vi "Main.vi"() -> ()   [LabVIEW 2019]
uses:
  support/Panel Selector (Radio Button).ctl
  support/Main_States.ctl
  support/Main_StateData.ctl
  Common Components/Hardware/DMM/DMM.lvclass
  Common Components/Hardware/FGEN/Function Generator.lvclass
  Common Components/Hardware/Scope/Scope.lvclass
panel:
  in  "Panel Selector (Radio Button)":T1
  # "Componentized Demo"
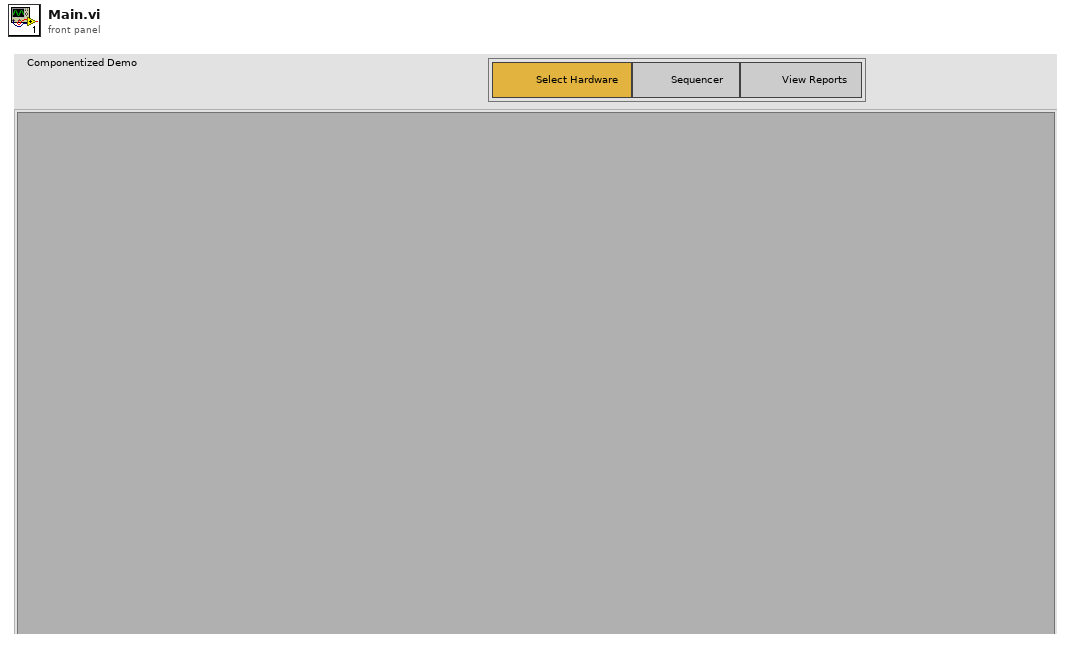
[diagram p1: front panel]
types:
  T1 = typedef "Panel Selector (Radio Button).ctl" = enum32{"Select HW", "Sequencer", "View Reports"}
  T2 = typedef "Main_StateData.ctl" = cluster{"Subpanel VI refs":refnum<vi>[]}
  T3 = typedef "Main_States.ctl" = enum16{"Initialize", "Wait for Event", "Shutdown"}
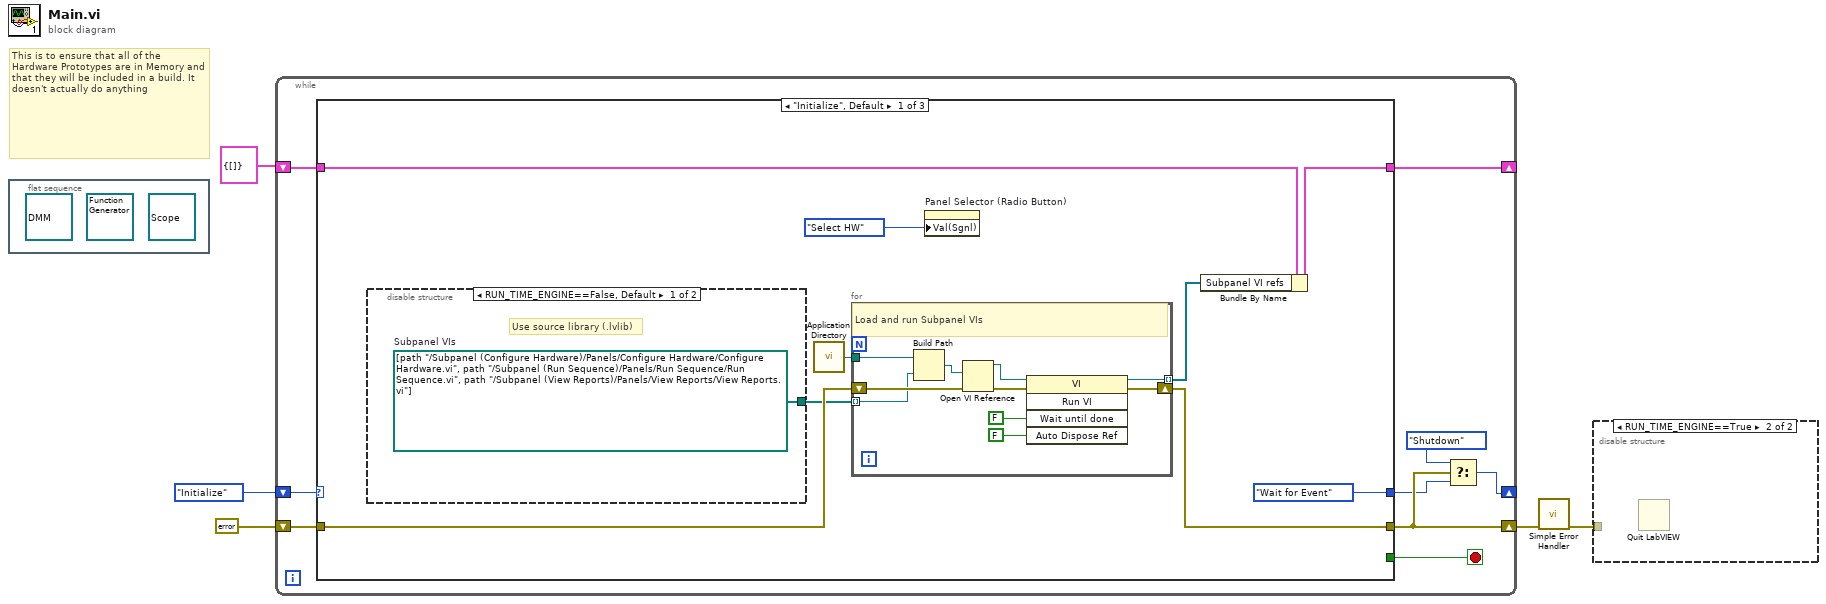
[diagram p0: block diagram]
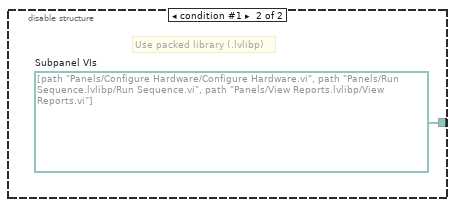
[diagram p3: hidden frame]
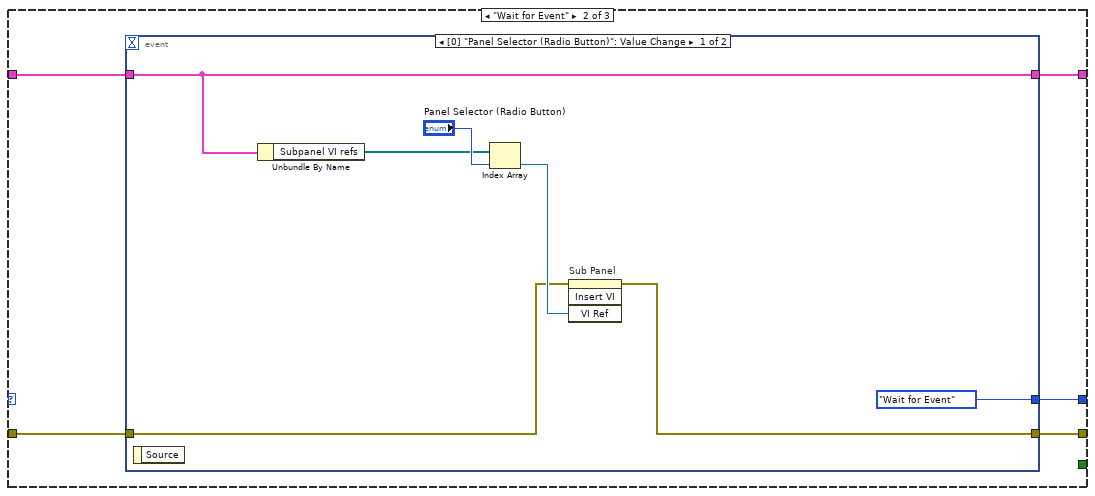
[diagram p4: hidden frame]
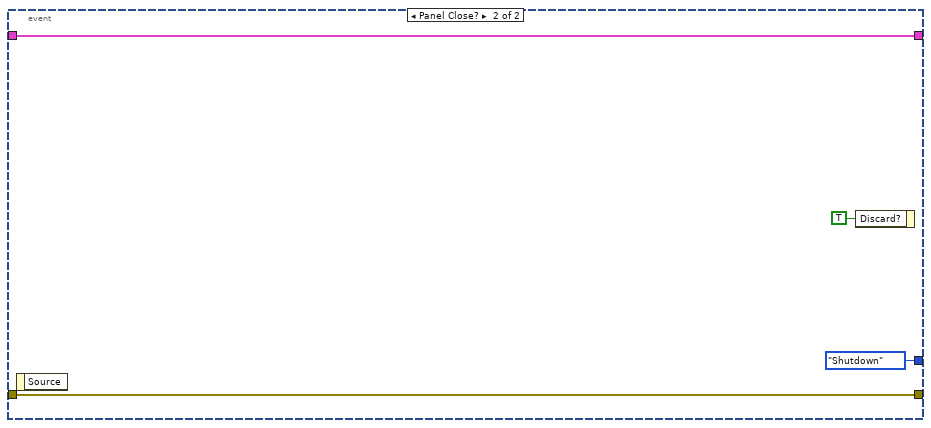
[diagram p5: hidden frame]
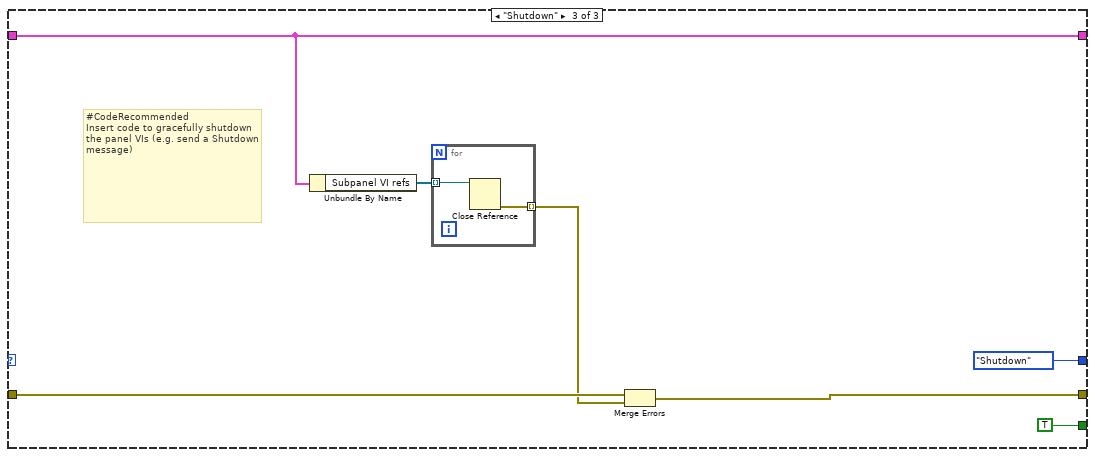
[diagram p6: hidden frame]
diagram:
  # "This is to ensure that all of the Hardware Prototypes are in Memory and that they will be included in a build. It doesn't actually do anything"
  n1 = flat-sequence {
    frame #0 {
      (unwired) refnum<class "Scope.lvclass"> refnum ("Hardware.lvlib:Scope.lvclass")
      (unwired) refnum<class "Function Generator.lvclass"> refnum ("Hardware.lvlib:Function Generator.lvclass")
      (unwired) refnum<class "DMM.lvclass"> refnum ("Hardware.lvlib:DMM.lvclass")
    }
  }
  n2 = while {
    shift-right: [w6] -> _
    shift-left: Main_States."Initialize" -> [w14]
    shift-right: [w9] -> w2
    shift-left: errorcluster {"status"=FALSE, "code"=0, "source"=""} ("error constant") -> [w12]
    shift-right: [w10] -> _
    shift-left: T2 {"Subpanel VI refs"=[]} ("Main_StateData") -> [w11]
    stop <- w13 stop-if-true
    n3 = case shown="\"Initialize\", Default" w14 {
      tunnel: [Main_States."Wait for Event" w40 Main_States."Shutdown"] -> w8
      tunnel: [_ _ TRUE] -> w13
      tunnel: w12 -> [w21 w37 w56]
      tunnel: [w20 w36 w53] -> w9
      tunnel: w11 -> [w18 w39 w55]
      tunnel: [w17 w38 w55] -> w10
      frame "Initialize", Default {
        n4 = disable-structure shown="RUN_TIME_ENGINE==False, Default" {
          disable-tunnel: [w24 w25] -> w19
          frame condition #0 (active) {
            w24 = path[] [path "../Subpanel (Configure Hardware)/Panels/Configure Hardware/Configure Hardware.vi", path "../Subpanel (Run Sequence)/Panels/Run Sequence/Run Sequence.vi", path "../Subpanel (View Reports)/Panels/View Reports/View Reports.vi"]  # Subpanel VIs
            # "Use source library (.lvlib)"
          }
          frame condition #1 {
            w25 = path[] [path "Panels/Configure Hardware/Configure Hardware.vi", path "Panels/Run Sequence.lvlibp/Run Sequence.vi", path "Panels/View Reports.lvlibp/View Reports.vi"]  # Subpanel VIs
            # "Use packed library (.lvlibp)"
          }
        }
        n5 = call <vilib>:"Application Directory.vi"() -> ("Application Directory"=w23:path)
        n6 = for {
          tunnel: [w31] -> w16 mode=indexing
          shift-right: [w29] -> w20
          shift-left: w21 -> [w30]
          tunnel: w23 -> [w28]
          tunnel: w19 -> [w26] mode=indexing
          # "Load and run Subpanel VIs"
          n7 = Build Path(base path=w28, name or relative path=w26) -> (appended path=w27:path)
          n8 = Open VI Reference(vi path=w27, error in (no error)=w30) -> (vi reference=w32:refnum<vi>, error out=w33:errorcluster)  [unwired: 4 in]
          n9 = invoke class="VI" method="Run VI"(reference=w32, error in=w33, "Wait until done"=FALSE ("Wait Until Done"), "Auto Dispose Ref"=FALSE ("Auto Dispose Reference")) -> (reference out=w31:refnum<vi>, error out=w29:errorcluster)  [unwired: 1 in, 3 out]
        }
        n10 = property on="Panel Selector (Radio Button)" class="RadioBtnsControl (strict)"("Val(Sgnl)"=Panel_Selector_(Radio_Button)."Select HW" ("Value (Signaling)")) -> ()  [unwired: 2 in, 2 out]
        n11 = Bundle By Name(cluster=w18, "Subpanel VI refs"=w16) -> (w17:T2)
      }
      frame "Wait for Event" {
        n12 = event shown="[0] \"Panel Selector (Radio Button)\": Value Change" {
          selector: _ -> [_ _]
          dyn-events: _ -> [_ _]
          timeout: _ -> [_ _]
          tunnel: [Main_States."Wait for Event" Main_States."Shutdown"] -> w40
          tunnel: w39 -> [w45 w49]
          tunnel: [w45 w49] -> w38
          tunnel: w37 -> [w42 w48]
          tunnel: [w41 w48] -> w36
          event Value Change {
            n13 = event-data() -> ()  [unwired: 1 in, 1 out]
            n14 = Unbundle By Name(w45) -> ("Subpanel VI refs"=w44:refnum<vi>[])
            n15 = Index Array(array=w44, index="Panel Selector (Radio Button)") -> (element=w43:refnum<vi>)
            n16 = invoke on="Sub Panel" class="SubPnl" method="Insert VI"(error in=w42, "VI Ref"=w43) -> (error out=w41:errorcluster)  [unwired: 2 in, 3 out]
          }
          event Panel Close? {
            n17 = event-data() -> ()  [unwired: 1 in, 1 out]
            n18 = event-data("Discard?"=TRUE) -> ()  [unwired: 1 in, 1 out]
          }
        }
      }
      frame "Shutdown" {
        # "#CodeRecommended\nInsert code to gracefully shutdown the panel VIs (e.g. send a Shutdown message)"
        n19 = Unbundle By Name(w55) -> ("Subpanel VI refs"=w54:refnum<vi>[])
        n20 = for {
          tunnel: w54 -> [w60] mode=indexing
          tunnel: [w59] -> w52 mode=indexing
          n21 = Close Reference(reference=w60) -> (error out=w59:errorcluster)  [unwired: 1 in]
        }
        n22 = Merge Errors(w56, w52) -> (w53:errorcluster)
      }
    }
    n23 = Select(t=Main_States."Shutdown", s=w9, f=w8) -> (s? t:f=w6:T3)
  }
  n24 = call <vilib>:"Simple Error Handler.vi"("error in (no error)"=w2) -> ("error out"=w1:errorcluster)  [unwired: 4 in, 4 out]
  n25 = disable-structure shown="RUN_TIME_ENGINE==True" {
    disable-tunnel: w1 -> [_ _]
    frame condition #0 (active) {
    }
    frame condition #1 {
      n26 = Quit LabVIEW() -> ()  [unwired: 1 in]
    }
  }
